vi "FPGA-Programm-11-15.vi"() -> ()   [LabVIEW 2010]
uses:
  markus/version feb 2012/gvboolesch.vi
  <vilib>/eio/EIONode/EIONode.xnode
  <vilib>/LabVIEW Targets/FPGA/cRIO/shared/nicrio_ModuleControls/nicrio_cRIO-9871_FlowControlEnum.ctl
  <vilib>/LabVIEW Targets/FPGA/cRIO/shared/nicrio_ModuleControls/nicrio_cRIO-9871_StopBitsEnum.ctl
  <vilib>/LabVIEW Targets/FPGA/cRIO/shared/nicrio_ModuleControls/nicrio_cRIO-9871_ParityEnum.ctl
  <vilib>/LabVIEW Targets/FPGA/cRIO/shared/nicrio_ModuleControls/nicrio_cRIO-9871_DataBitsEnum.ctl
  <vilib>/LabVIEW Targets/FPGA/cRIO/shared/nicrio_ModuleControls/nicrio_cRIO-9871_BaudRateEnum.ctl
panel:
  in  "LHPulse(us)":T1
  in  "LHHeizen?":T2
  in  "USetp[V]MainMach2":fxp<+/-,16,4> format="%.14g"
  in  "USetp[V]MainMach1":fxp<+/-,16,4> format="%.14g"
  in  "Umax[V]MainMach2":fxp<+/-,16,4> format="%.14g"
  in  "Umax[V]MainMach1":fxp<+/-,16,4> format="%.14g"
  in  "PIDMainMach2":T3 {"proportional gain (Kc)" format="%.11g"; "integral gain (Kc*Ts/Ti)" format="%.11g"; "derivative gain (Kc*Td/Ts)" format="%.11g"}
  in  "PIDMainMach1":T3 {"proportional gain (Kc)" format="%.11g"; "integral gain (Kc*Ts/Ti)" format="%.11g"; "derivative gain (Kc*Td/Ts)" format="%.11g"}
  in  "Heizen?MainMach2":bool
  in  "Heizen?MainMach1":bool
  out "U[V]MainMach2":fxp<+/-,16,4> format="%.25g"
  out "U[V]MainMach1":fxp<+/-,16,4> format="%.25g"
  in  "Servo2An?":bool
  in  "Servo1An?":bool
  in  "Mod6/DIO":T4
  in  "Mod5/DIO":T5
  in  "USetp[V]PreMach2":fxp<+/-,16,4> format="%.14g"
  in  "USetp[V]PreMach1":fxp<+/-,16,4> format="%.14g"
  in  "Umax[V]PreMach2":fxp<+/-,16,4> format="%.14g"
  in  "Umax[V]PreMach1":fxp<+/-,16,4> format="%.14g"
  in  "PIDPreMach2":T3 {"proportional gain (Kc)" format="%.11g"; "integral gain (Kc*Ts/Ti)" format="%.11g"; "derivative gain (Kc*Td/Ts)" format="%.11g"}
  in  "PIDPreMach1":T3 {"proportional gain (Kc)" format="%.11g"; "integral gain (Kc*Ts/Ti)" format="%.11g"; "derivative gain (Kc*Td/Ts)" format="%.11g"}
  in  "UTempSPTrap2":fxp<+/-,16,4> format="%.14g"
  in  "UTempMaxTrap2":fxp<+/-,16,4> format="%.14g"
  in  "PIDTrap2":T3 {"proportional gain (Kc)" format="%.11g"; "integral gain (Kc*Ts/Ti)" format="%.11g"; "derivative gain (Kc*Td/Ts)" format="%.11g"}
  in  "UTempSPTrap1":fxp<+/-,16,4> format="%.14g"
  in  "UTempMaxTrap1":fxp<+/-,16,4> format="%.14g"
  in  "PIDTrap1":T3 {"proportional gain (Kc)" format="%.11g"; "integral gain (Kc*Ts/Ti)" format="%.11g"; "derivative gain (Kc*Td/Ts)" format="%.11g"}
  in  "Heizen?PreMach2":bool
  in  "Heizen?PreMach1":bool
  in  "Heizen?Trap2":bool
  in  "Heizen?Trap1":bool
  in  "ServosWarmHigh (us)KaltHigh(us)":T6
  in  "ServoTrap2kalt":bool
  in  "ServoTrap1kalt":bool
  in  "FIFO leer":bool
  in  "KonfigSeriell":T12
  in  "ServosPeriode(us)":u32=10
  out "U[V]PreMach1":fxp<+/-,16,4> format="%.25g"
  out "U[V]PreMach2":fxp<+/-,16,4> format="%.25g"
  in  "global stop":bool
  out "UTemp[V]Trap2":fxp<+/-,16,4> format="%.25g"
  out "UTemp[V]Trap1":fxp<+/-,16,4> format="%.25g"
  out "KonfigSeriellError":errorcluster
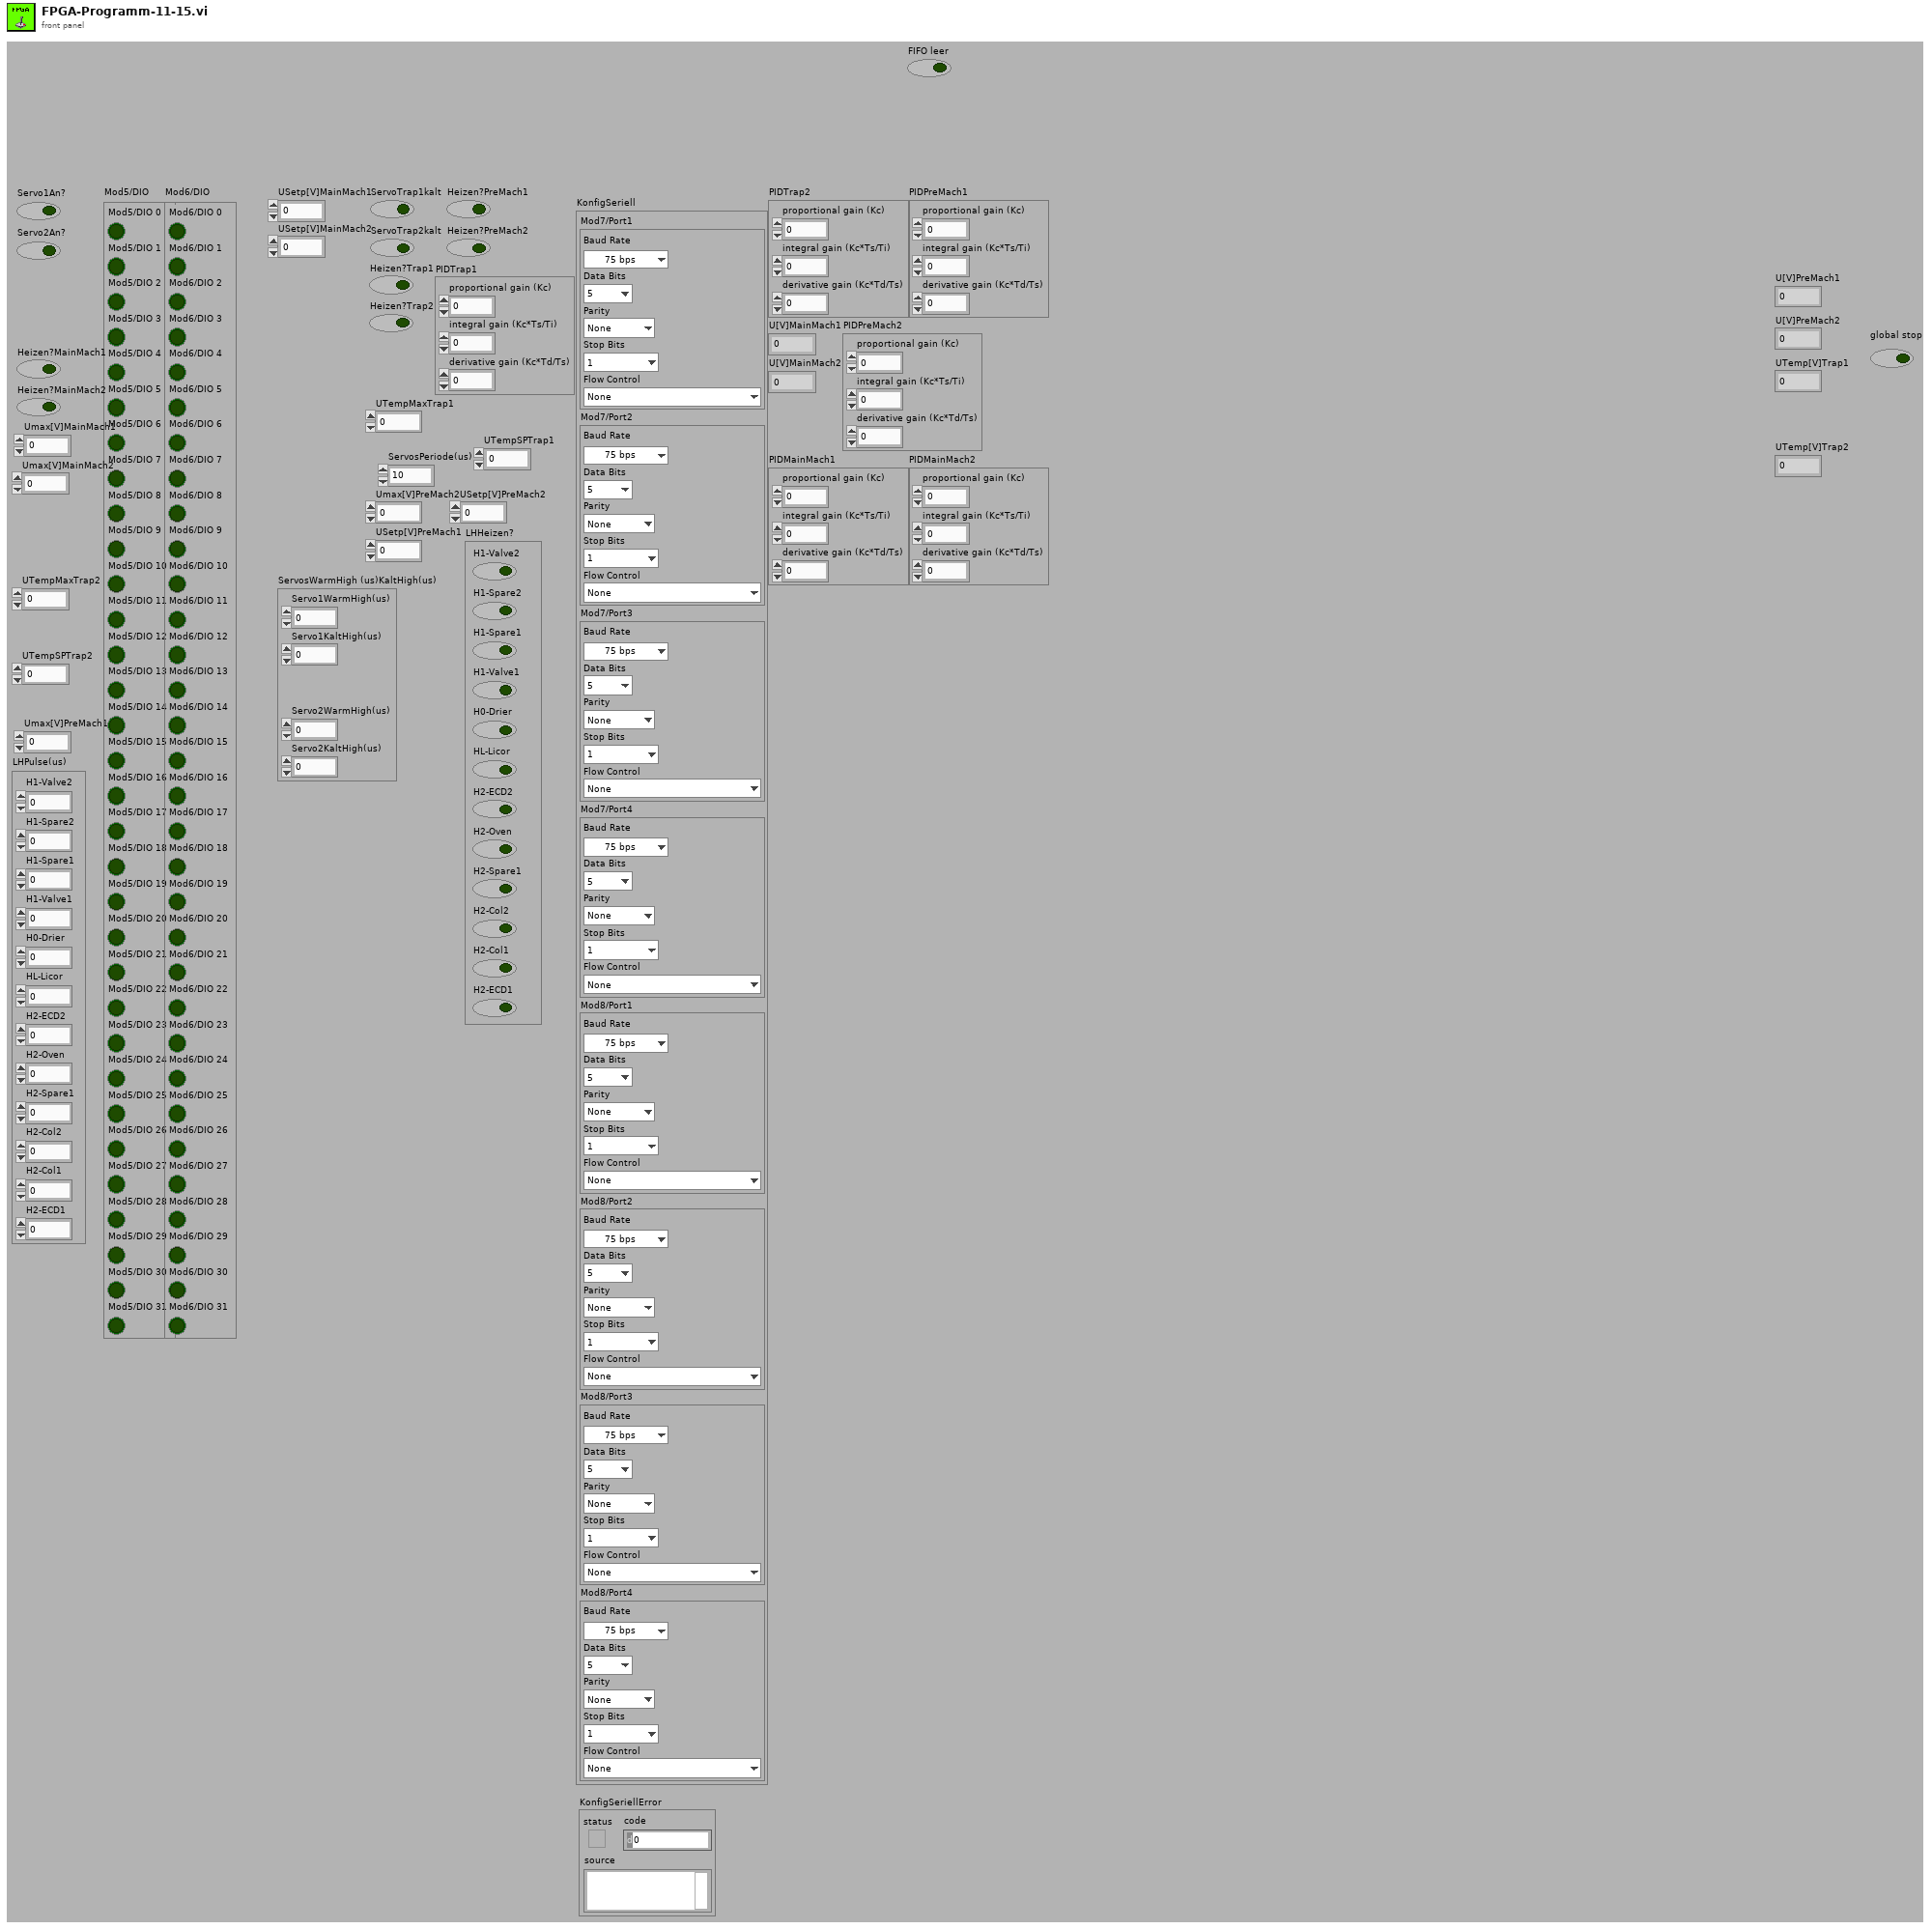
[diagram p1: front panel]
types:
  T1 = cluster{"H1-Valve2":u32, "H1-Spare2":u32, "H1-Spare1":u32, "H1-Valve1":u32, "H0-Drier":u32, "HL-Licor":u32, "H2-ECD2":u32, "H2-Oven":u32, "H2-Spare1":u32, "H2-Col2":u32, "H2-Col1":u32, "H2-ECD1":u32}
  T2 = cluster{"H1-Valve2":bool, "H1-Spare2":bool, "H1-Spare1":bool, "H1-Valve1":bool, "H0-Drier":bool, "HL-Licor":bool, "H2-ECD2":bool, "H2-Oven":bool, "H2-Spare1":bool, "H2-Col2":bool, "H2-Col1":bool, "H2-ECD1":bool}
  T3 = cluster{"proportional gain (Kc)":fxp<+/-,16,8>, "integral gain (Kc*Ts/Ti)":fxp<+/-,16,8>, "derivative gain (Kc*Td/Ts)":fxp<+/-,16,8>}
  T4 = cluster{"Mod6/DIO 0":bool, "Mod6/DIO 1":bool, "Mod6/DIO 2":bool, "Mod6/DIO 3":bool, "Mod6/DIO 4":bool, "Mod6/DIO 5":bool, "Mod6/DIO 6":bool, "Mod6/DIO 7":bool, "Mod6/DIO 8":bool, "Mod6/DIO 9":bool, "Mod6/DIO 10":bool, "Mod6/DIO 11":bool, "Mod6/DIO 12":bool, "Mod6/DIO 13":bool, "Mod6/DIO 14":bool, "Mod6/DIO 15":bool, "Mod6/DIO 16":bool, "Mod6/DIO 17":bool, "Mod6/DIO 18":bool, "Mod6/DIO 19":bool, "Mod6/DIO 20":bool, "Mod6/DIO 21":bool, "Mod6/DIO 22":bool, "Mod6/DIO 23":bool, "Mod6/DIO 24":bool, "Mod6/DIO 25":bool, "Mod6/DIO 26":bool, "Mod6/DIO 27":bool, "Mod6/DIO 28":bool, "Mod6/DIO 29":bool, "Mod6/DIO 30":bool, "Mod6/DIO 31":bool}
  T5 = cluster{"Mod5/DIO 0":bool, "Mod5/DIO 1":bool, "Mod5/DIO 2":bool, "Mod5/DIO 3":bool, "Mod5/DIO 4":bool, "Mod5/DIO 5":bool, "Mod5/DIO 6":bool, "Mod5/DIO 7":bool, "Mod5/DIO 8":bool, "Mod5/DIO 9":bool, "Mod5/DIO 10":bool, "Mod5/DIO 11":bool, "Mod5/DIO 12":bool, "Mod5/DIO 13":bool, "Mod5/DIO 14":bool, "Mod5/DIO 15":bool, "Mod5/DIO 16":bool, "Mod5/DIO 17":bool, "Mod5/DIO 18":bool, "Mod5/DIO 19":bool, "Mod5/DIO 20":bool, "Mod5/DIO 21":bool, "Mod5/DIO 22":bool, "Mod5/DIO 23":bool, "Mod5/DIO 24":bool, "Mod5/DIO 25":bool, "Mod5/DIO 26":bool, "Mod5/DIO 27":bool, "Mod5/DIO 28":bool, "Mod5/DIO 29":bool, "Mod5/DIO 30":bool, "Mod5/DIO 31":bool}
  T6 = cluster{"Servo1WarmHigh(us)":u32, "Servo1KaltHigh(us)":u32, "Servo2WarmHigh(us)":u32, "Servo2KaltHigh(us)":u32}
  T7 = typedef "nicrio_cRIO-9871_BaudRateEnum.ctl" = enum16{"75 bps", "110 bps", "134 bps", "150 bps", "300 bps", "600 bps", "1200 bps", "1800 bps", "2400 bps", "4800 bps", "7200 bps", "9600 bps", "14.4 kbps", "19.2 kbps", "28.8 kbps", "38.4 kbps", "57.6 kbps", "115.2 kbps", "230.4 kbps", "460.8 kbps", "921.6 kbps"}
  T8 = typedef "nicrio_cRIO-9871_DataBitsEnum.ctl" = enum8{"5", "6", "7", "8"}
  T9 = typedef "nicrio_cRIO-9871_ParityEnum.ctl" = enum8{"None", "Odd", "Even", "Mark", "Space"}
  T10 = typedef "nicrio_cRIO-9871_StopBitsEnum.ctl" = enum8{"1", "1.5", "2"}
  T11 = typedef "nicrio_cRIO-9871_FlowControlEnum.ctl" = enum8{"None", "Software (XON / XOFF)", "Hardware (RTS / CTS)"}
  T12 = cluster{"Mod7/Port1":cluster{"Baud Rate":T7, "Data Bits":T8, "Parity":T9, "Stop Bits":T10, "Flow Control":T11}, "Mod7/Port2":cluster{"Baud Rate":T7, "Data Bits":T8, "Parity":T9, "Stop Bits":T10, "Flow Control":T11}, "Mod7/Port3":cluster{"Baud Rate":T7, "Data Bits":T8, "Parity":T9, "Stop Bits":T10, "Flow Control":T11}, "Mod7/Port4":cluster{"Baud Rate":T7, "Data Bits":T8, "Parity":T9, "Stop Bits":T10, "Flow Control":T11}, "Mod8/Port1":cluster{"Baud Rate":T7, "Data Bits":T8, "Parity":T9, "Stop Bits":T10, "Flow Control":T11}, "Mod8/Port2":cluster{"Baud Rate":T7, "Data Bits":T8, "Parity":T9, "Stop Bits":T10, "Flow Control":T11}, "Mod8/Port3":cluster{"Baud Rate":T7, "Data Bits":T8, "Parity":T9, "Stop Bits":T10, "Flow Control":T11}, "Mod8/Port4":cluster{"Baud Rate":T7, "Data Bits":T8, "Parity":T9, "Stop Bits":T10, "Flow Control":T11}}
  T13 = cluster{"Per[us]Trap1":u32, "warten[us]Trap1":u32, "Per[us]Trap2":u32, "warten[us]Trap2":u32, "Per[us]Mach":u16, "vor der Messung [us]Mach":u16, "wie viele Messwerte?Mach":u16, "Abstand zwischen Messungen [us]Mach":u16}
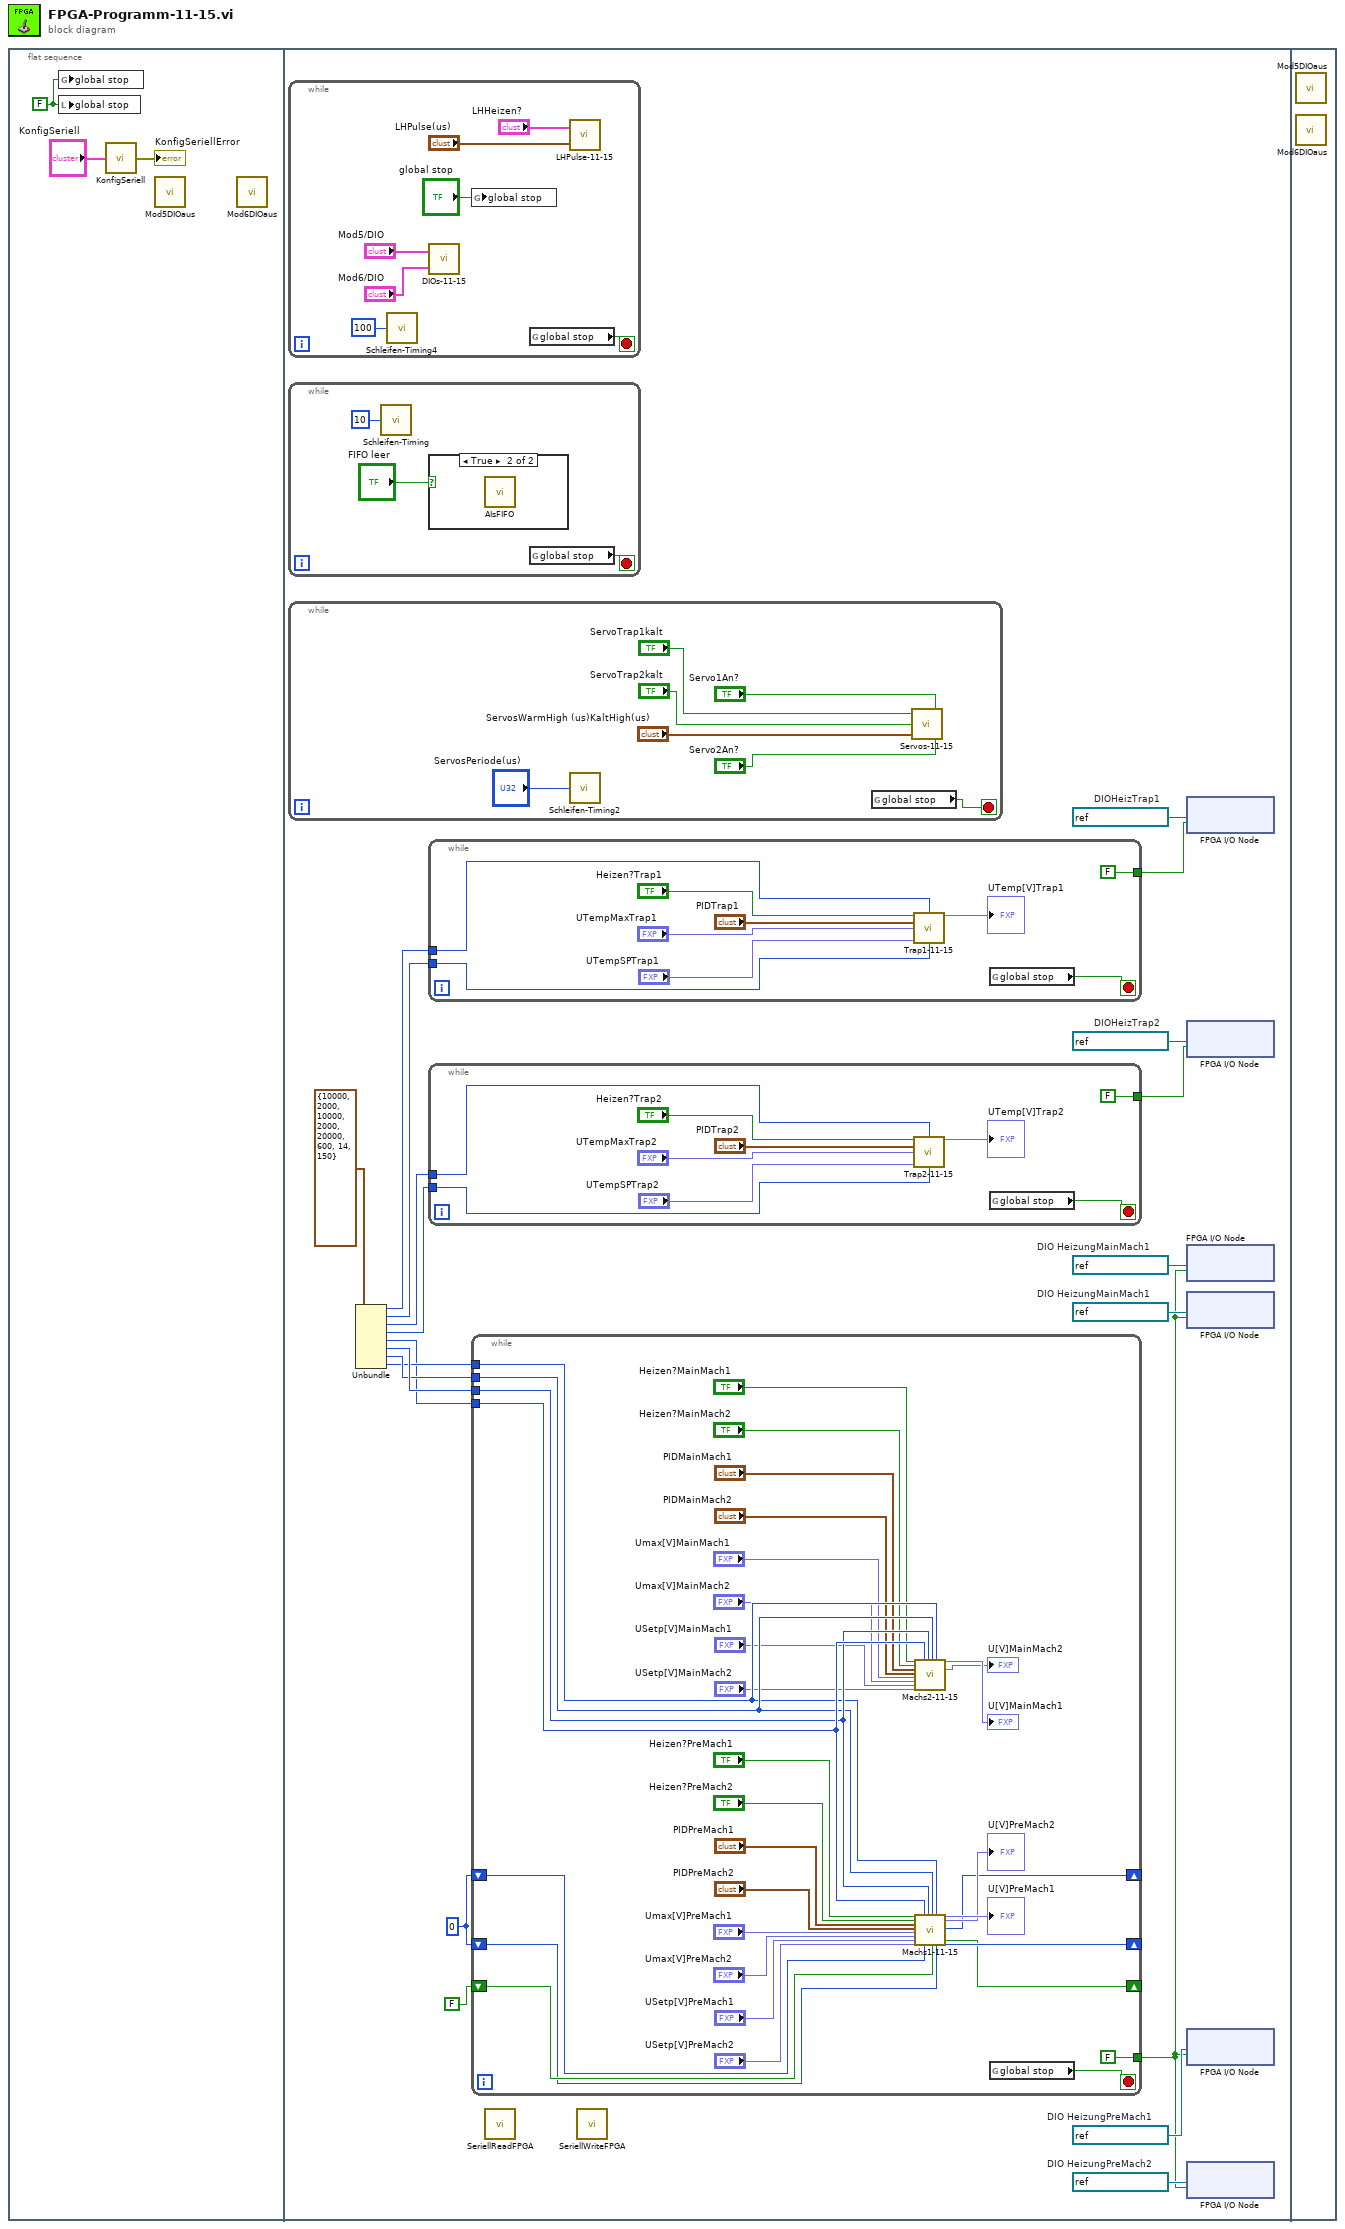
[diagram p0: block diagram]
diagram:
  n1 = flat-sequence {
    frame #0 {
      w1 = FALSE
      n2 = global write "gvboolesch.vi" "global stop"(w1) -> ()
      n3 = local write "global stop"(w1) -> ()
      n4 = call "KonfigSeriell.vi"("KonfigSeriell"="KonfigSeriell") -> ("KonfigSeriell"=→"KonfigSeriellError":errorcluster)
      n5 = call "Mod5DIOaus.vi"() -> ()  [unwired: 1 in]
      n6 = call "Mod6DIOaus.vi"() -> ()  [unwired: 1 in]
    }
    frame #1 {
      w9 = refnum<k21> "Mod6/DIO17"  # DIO HeizungMainMach1
      w10 = refnum<k21> "Mod6/DIO28"  # DIO HeizungMainMach1
      w18 = refnum<k21> "Mod6/DIO22"  # DIO HeizungPreMach2
      w19 = refnum<k21> "Mod6/DIO23"  # DIO HeizungPreMach1
      w21 = refnum<k21> "Mod6/DIO18"  # DIOHeizTrap2
      w23 = refnum<k21> "Mod6/DIO19"  # DIOHeizTrap1
      w6 = u16 0
      n7 = while {
        stop <- w31 stop-if-true
        n8 = call "Schleifen-Timing4"("Count(mSec)"=u8 100) -> ()  [unwired: 1 out]
        n9 = call "DIOs-11-15.vi"("Mod6/DIOs"="Mod6/DIO", "Mod5/DIOs"="Mod5/DIO") -> ()  [unwired: 3 in]
        n10 = global write "gvboolesch.vi" "global stop"("global stop") -> ()
        n11 = global read "gvboolesch.vi" "global stop"() -> (w31:bool)
        n12 = call "LHPulse-11-15.vi"("LHPulse(us)"="LHPulse(us)", "LHHeizen?"="LHHeizen?") -> ()  [unwired: 2 in]
      }
      n13 = while {
        stop <- w26 stop-if-true
        n14 = call "Schleifen-Timing"("Count(mSec)"=u8 10) -> ()  [unwired: 1 out]
        n15 = case shown="True" "FIFO leer" {
          frame False {
          }
          frame True {
            n16 = call "AIsFIFO.vi"() -> ()  [unwired: 12 in]
          }
        }
        n17 = global read "gvboolesch.vi" "global stop"() -> (w26:bool)
      }
      n18 = while {
        stop <- w72 stop-if-true
        n19 = call "Schleifen-Timing2"("Count(uSec)"="ServosPeriode(us)") -> ()  [unwired: 1 out]
        n20 = global read "gvboolesch.vi" "global stop"() -> (w72:bool)
        n21 = call "Servos-11-15.vi"("Servo2An?"="Servo2An?", "Servo1An?"="Servo1An?", "ServosWarmHigh (us)KaltHigh(us)"="ServosWarmHigh (us)KaltHigh(us)", "ServoTrap2kalt"="ServoTrap2kalt", "ServoTrap1kalt"="ServoTrap1kalt") -> ()
      }
      n22 = Unbundle(T13 {"Per[us]Trap1"=10000, "warten[us]Trap1"=2000, "Per[us]Trap2"=10000, "warten[us]Trap2"=2000, "Per[us]Mach"=20000, "vor der Messung [us]Mach"=600, "wie viele Messwerte?Mach"=14, "Abstand zwischen Messungen [us]Mach"=150} ("SHFest")) -> ("Per[us]Trap1"=w14:u32, "warten[us]Trap1"=w13:u32, "Per[us]Trap2"=w12:u32, "warten[us]Trap2"=w11:u32, "Per[us]Mach"=w5:u16, "vor der Messung [us]Mach"=w17:u16, "wie viele Messwerte?Mach"=w16:u16, "Abstand zwischen Messungen [us]Mach"=w15:u16)
      n23 = while {
        tunnel: [FALSE ("I/O Item")] -> w22
        tunnel: w14 -> [w84]
        tunnel: w13 -> [w83]
        stop <- w90 stop-if-true
        n24 = call "Trap1-11-15.vi"("Heizen?Trap1"="Heizen?Trap1", "Per[us]Trap1"=w84, "PIDTrap1"="PIDTrap1", "UTempMaxTrap1"="UTempMaxTrap1", "UTempSPTrap1"="UTempSPTrap1", "warten[us]Trap1"=w83) -> ("UTemp[V]Trap1"=→"UTemp[V]Trap1":fxp<+/-,16,4>)  [unwired: 9 in]
        n25 = global read "gvboolesch.vi" "global stop"() -> (w90:bool)
      }
      n26 = while {
        tunnel: [FALSE ("I/O Item")] -> w20
        tunnel: w12 -> [w79]
        tunnel: w11 -> [w78]
        stop <- w81 stop-if-true
        n27 = call "Trap2-11-15.vi"("Heizen?Trap2"="Heizen?Trap2", "Per[us]Trap2"=w79, "PIDTrap2"="PIDTrap2", "UTempMaxTrap2"="UTempMaxTrap2", "UTempSPTrap2"="UTempSPTrap2", "warten[us]Trap2"=w78) -> ("UTemp[V]Trap2"=→"UTemp[V]Trap2":fxp<+/-,16,4>)  [unwired: 9 in]
        n28 = global read "gvboolesch.vi" "global stop"() -> (w81:bool)
      }
      n29 = while {
        shift-right: [w57] -> _
        shift-left: w6 -> [w54]
        shift-right: [w56] -> _
        shift-left: FALSE -> [w55]
        tunnel: [FALSE] -> w8
        tunnel: w5 -> [w47]
        tunnel: w17 -> [w46]
        tunnel: w16 -> [w45]
        tunnel: w15 -> [w44]
        shift-right: [w49] -> _
        shift-left: w6 -> [w48]
        stop <- w65 stop-if-true
        n30 = call "Machs2-11-15.vi"("Heizen?Mach1"="Heizen?MainMach1", "Heizen?Mach2"="Heizen?MainMach2", "PIDMach1"="PIDMainMach1", "PIDMach2"="PIDMainMach2", "Umax[V]Mach1"="Umax[V]MainMach1", "Umax[V]Mach2"="Umax[V]MainMach2", "USetp[V]Mach1"="USetp[V]MainMach1", "USetp[V]Mach2"="USetp[V]MainMach2", "Per[us]Mach"=w47, "vor der Messung [us]Mach"=w46, "wie viele Messwerte?Mach"=w45, "Abstand zwischen Messungen [us]Mach"=w44) -> ("U[V]Mach1"=→"U[V]MainMach1":fxp<+/-,16,4>, "U[V]Mach2"=→"U[V]MainMach2":fxp<+/-,16,4>)  [unwired: 14 in]
        n31 = call "Machs1-11-15.vi"("Heizen?Mach1"="Heizen?PreMach1", "Heizen?Mach2"="Heizen?PreMach2", "PIDMach1"="PIDPreMach1", "PIDMach2"="PIDPreMach2", "Umax[V]Mach1"="Umax[V]PreMach1", "Umax[V]Mach2"="Umax[V]PreMach2", "USetp[V]Mach1"="USetp[V]PreMach1", "USetp[V]Mach2"="USetp[V]PreMach2", "Per[us]Mach"=w47, "Mach1maxHigh"=w48, "vor der Messung [us]Mach"=w46, "wie viele Messwerte?Mach"=w45, "Mach2High?"=w55, "Abstand zwischen Messungen [us]Mach"=w44, "Mach2High"=w54) -> ("U[V]Mach1"=→"U[V]PreMach1":fxp<+/-,16,4>, "U[V]Mach2"=→"U[V]PreMach2":fxp<+/-,16,4>, "Mach1maxHigh"=w49:u16, "Mach2High?"=w56:bool, "Mach2High"=w57:u16)  [unwired: 8 in]
        n32 = global read "gvboolesch.vi" "global stop"() -> (w65:bool)
      }
      n33 = call "SeriellReadFPGA.vi"() -> ()  [unwired: 12 in]
      n34 = call "SeriellWriteFPGA.vi"() -> ()  [unwired: 12 in]
      n35 = xnode "FPGA I/O Node"("I/O Item"=w22, "FPGA I/O In"=w23) -> ()  [unwired: 1 out]
      n36 = xnode "FPGA I/O Node"("I/O Item"=w20, "FPGA I/O In"=w21) -> ()  [unwired: 1 out]
      n37 = xnode "FPGA I/O Node"("I/O Item"=w8, "FPGA I/O In"=w9) -> ()  [unwired: 1 out]
      n38 = xnode "FPGA I/O Node"("I/O Item"=w8, "FPGA I/O In"=w10) -> ()  [unwired: 1 out]
      n39 = xnode "FPGA I/O Node"("I/O Item"=w8, "FPGA I/O In"=w19) -> ()  [unwired: 1 out]
      n40 = xnode "FPGA I/O Node"("I/O Item"=w8, "FPGA I/O In"=w18) -> ()  [unwired: 1 out]
    }
    frame #2 {
      n41 = call "Mod5DIOaus.vi"() -> ()  [unwired: 1 in]
      n42 = call "Mod6DIOaus.vi"() -> ()  [unwired: 1 in]
    }
  }
